vi "OEE_PULSE_is_it_time_for_next_pulse.vi"(11 "last_pulse":timestamp) -> (3 "next_state":T1)   [LabVIEW 2019]
uses:
  OEE_PULSE_sequence_state.ctl
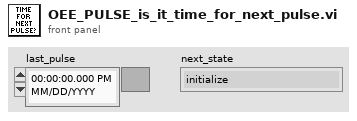
[diagram p1: front panel]
types:
  T1 = typedef "OEE_PULSE_sequence_state.ctl" = enum16{"initialize", "get_next_state", "start_pulses", "stop_pulses", "pulse", "error", "stop"}
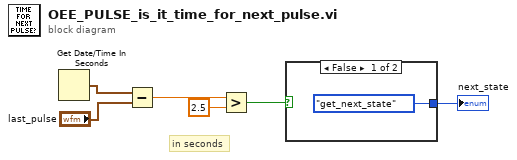
[diagram p0: block diagram]
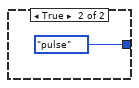
[diagram p2: hidden frame]
diagram:
  # "in seconds"
  n1 = Get Date/Time In Seconds() -> (seconds since 1Jan1904=w1:timestamp)
  n2 = Subtract(x=w1, y="last_pulse") -> (x-y=w5:dbl)
  n3 = Greater?(x=w5, y=2.5) -> (0:w3:bool)
  n4 = case shown="False" w3 {
    tunnel: [OEE_PULSE_sequence_state."get_next_state" ("state") OEE_PULSE_sequence_state."pulse" ("state")] -> w6
    frame False {
    }
    frame True {
    }
  }
  "next_state" <- w6
